vi "ReadAxisHomedState.vi"(8 "error in (no error)":errorcluster, 9 "Axis (1..4)":T1=1 items=["X"=1, "Y"=2, "Z"=3, "T"=4], 11 "VXMx2 in":refnum<class "VXMx2.lvclass">) -> (0 "error out":errorcluster, 1 "Homed=T":bool, 3 "VXMx2 out":refnum<class "VXMx2.lvclass">)   [LabVIEW 2018, in "VXMx2.lvclass"]
uses:
  VXMx2.lvclass
  <instrlib>/Velmex VXM/Public/VXM Axis.ctl
  VXMx2.lvclass/VXMx2.ctl
  <instrlib>/Velmex VXM/Velmex VXM.lvlib
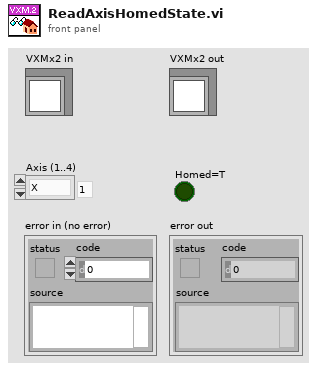
[diagram p1: front panel]
types:
  T1 = typedef "Velmex VXM.lvlib/VXM Axis.ctl" = u16
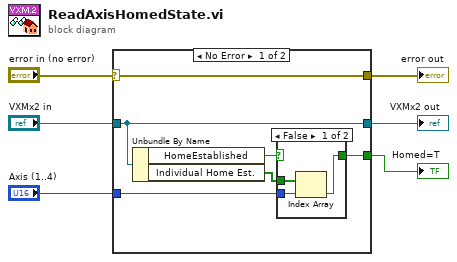
[diagram p0: block diagram]
diagram:
  n1 = case shown="No Error" "error in (no error)" {
    selector: "error in (no error)" -> [w12 w18]
    tunnel: [w12 w18] -> w5
    tunnel: [w11 w17] -> w3
    tunnel: "VXMx2 in" -> [w11 w17]
    tunnel: [w9 _] -> w2
    tunnel: "Axis (1..4)" -> [w7 _]
    frame No Error {
      n2 = Unbundle By Name(w11) -> ("HomeEstablished"=w10:bool, "Individual Home Est."=w8:bool[])
      n3 = case shown="False" w10 {
        selector: w10 -> [_ w16]
        tunnel: [w13 w16] -> w9
        tunnel: w8 -> [w15 _]
        tunnel: w7 -> [w14 _]
        frame False {
          n4 = Index Array(array=w15, index=w14) -> (element=w13:bool)
        }
        frame True {
        }
      }
    }
    frame Error {
    }
  }
  "error out" <- w5
  "VXMx2 out" <- w3
  "Homed=T" <- w2
